vi "TRG_SOURCE - Type.vi"(8 "error in (no error)":errorcluster, 11 "TRG_SOURCE":T1) -> (0 "error out":errorcluster, 3 "TRG_SOURCE_VALUE":i32)   [LabVIEW 2015]
doc: "<b>Trigger Source settings.</b>\nOFF : Camera works in free run mode.\nEDGE_RISING : External trigger (rising edge).\nEDGE_FALLING : External trigger (falling edge).\nSOFTWARE : Software(manual) trigger."
uses:
  C:/GIT/Cameras3.x/Integrations/Labview/xiLib/xiLIB_32bit/xiLIB/xiCamLib/API/x86/xiApi.NET.dll
  xiLIB_32bit/xiLIB/xiCamLib/API/x86/xiApi.NET.dll
  TRG_SOURCE.ctl
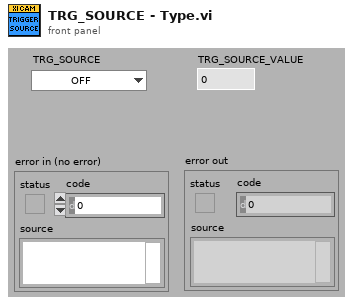
[diagram p1: front panel]
types:
  T1 = typedef "TRG_SOURCE.ctl" = enum16{"OFF", "EDGE_RISING", "EDGE_FALLING", "SOFTWARE"}
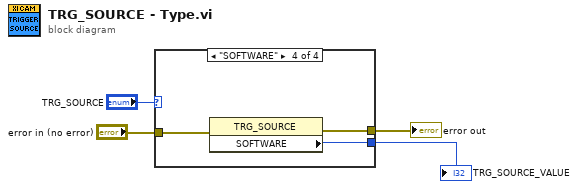
[diagram p0: block diagram]
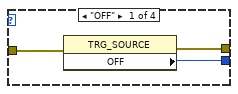
[diagram p2: hidden frame]
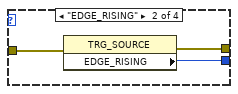
[diagram p3: hidden frame]
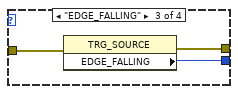
[diagram p4: hidden frame]
diagram:
  n1 = case shown="\"SOFTWARE\"" "TRG_SOURCE" {
    tunnel: "error in (no error)" -> [w7 w10 w13 w16]
    tunnel: [w6 w9 w12 w15] -> w2
    tunnel: [w5 w8 w11 w14] -> w1
    frame "OFF" {
      n2 = property class="TRG_SOURCE"(error in=w7) -> (error out=w6:errorcluster, "OFF"=w5:i32)  [unwired: 1 in, 1 out]
    }
    frame "EDGE_RISING" {
      n3 = property class="TRG_SOURCE"(error in=w10) -> (error out=w9:errorcluster, "EDGE_RISING"=w8:i32)  [unwired: 1 in, 1 out]
    }
    frame "EDGE_FALLING" {
      n4 = property class="TRG_SOURCE"(error in=w13) -> (error out=w12:errorcluster, "EDGE_FALLING"=w11:i32)  [unwired: 1 in, 1 out]
    }
    frame "SOFTWARE" {
      n5 = property class="TRG_SOURCE"(error in=w16) -> (error out=w15:errorcluster, "SOFTWARE"=w14:i32)  [unwired: 1 in, 1 out]
    }
  }
  "error out" <- w2
  "TRG_SOURCE_VALUE" <- w1
